vi "Get REF StringsAndValues.vi"(8 "error in (no error)":errorcluster, 11 "Channels.REF":T1 {"Roll-Off" min=1; "TC" min=0.0001 format="%#_3p"; "Phase" format="%.3g"; "Frequency" min=0.0001 max=10000.0 format="%.3g"; "Channel" min=1}) -> (0 "error out":errorcluster, 2 "REF Strings and Values":cluster{string, i32}[](array[cluster]))   [LabVIEW 2019, in "Instrument.Lockin.lvlib" / "Instrument UI.Lockin.lvclass"]
uses:
  Instrument UI.Lockin.lvclass
  Instrument.DAQ/Typedefs/REF.Channel--Cluster--Array.ctl
  Instrument.DAQ/Typedefs/REF.Channel--Cluster.ctl
  Instrument.DAQ/Instrument.DAQ.lvclass
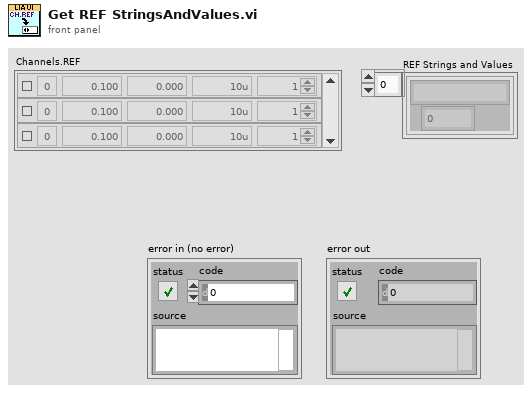
[diagram p1: front panel]
types:
  T1 = typedef "Instrument.Lockin.lvlib/Instrument.DAQ.lvclass/REF.Channel--Cluster--Array.ctl" = T2[]
  T2 = typedef "Instrument.Lockin.lvlib/Instrument.DAQ.lvclass/REF.Channel--Cluster.ctl" = cluster{"Enable?":bool, "Channel":i32, "Frequency":dbl, "Phase":dbl, "TC":dbl, "Roll-Off":i32}
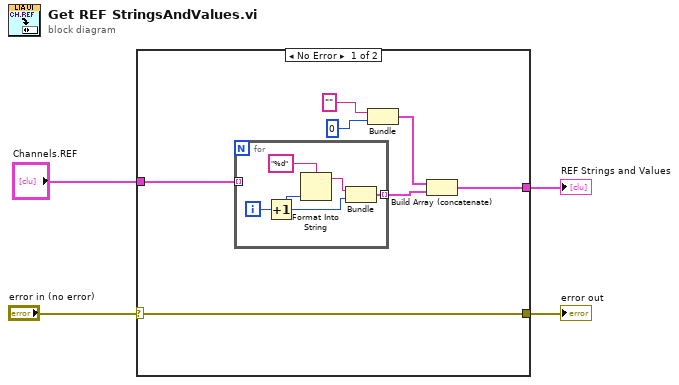
[diagram p0: block diagram]
diagram:
  n1 = case shown="No Error" "error in (no error)" {
    selector: "error in (no error)" -> [w11 w17]
    tunnel: [w7 _] -> w4
    tunnel: [w11 w17] -> w2
    tunnel: "Channels.REF" -> [w5 _]
    frame No Error {
      n2 = for {
        tunnel: [w15] -> w6 mode=indexing
        tunnel: w5 -> [_] mode=indexing
        i -> [w16]
        n3 = Increment(x=w16) -> (x+1=w14:i32)
        n4 = Format Into String(format string="%d", w14) -> (resulting string=w12:string)  [unwired: 2 in, 1 out]
        n5 = Bundle(w12, w14) -> (w15:cluster{string, i32})  [unwired: 1 in]
      }
      n6 = Bundle("format string"="", "x+1"=0) -> (w8:cluster{"format string":string, "x+1":i32})  [unwired: 1 in]
      n7 = Build Array (concatenate)(w8, w6) -> (w7:cluster{"format string":string, "x+1":i32}[])
    }
    frame Error {
    }
  }
  "REF Strings and Values" <- w4
  "error out" <- w2
